vi "Custom VISA Init Selector.vi"(5 "Interface filter (all)":T1={"GPIB"=TRUE, "Serial"=TRUE, "TCP"=TRUE, "USB"=TRUE}, 7 "Initial enumerate? (False)":bool, 8 "error in (no error)":errorcluster, 10 "VISA address (Empty)":refnum<visa-resource-name>, 11 "VISA menu ref":refnum<vi>) -> (0 "error out":errorcluster)   [LabVIEW 2020, in "Get COM Descriptor.lvlib"]
doc: "Call this to initialize custom VISA Ring control at start of panel. It will make initial menu with \"Refresh\" option. If you pass in VISA, it will make default item from the VISA address. Otherwise it will use Ring.Text as default.\nOptionally does initial VISA enumeration to fill in the Ring.\n\nDetails: https://github.com/smaslan/get-com-descriptor"
uses:
  Get COM Descriptor.lvlib
  Custom VISA Filters.ctl
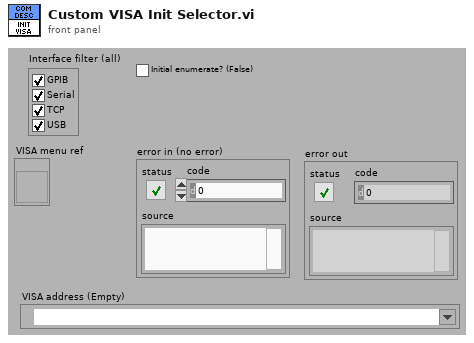
[diagram p1: front panel]
types:
  T1 = typedef "Get COM Descriptor.lvlib/Custom VISA Filters.ctl" = cluster{"GPIB":bool, "Serial":bool, "TCP":bool, "USB":bool}
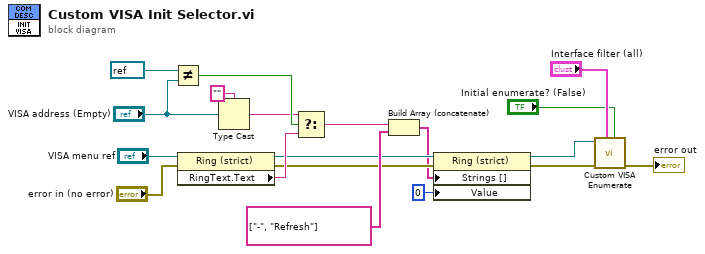
[diagram p0: block diagram]
diagram:
  n1 = Not Equal?(x=refnum<visa-resource-name> refnum ("reference"), y="VISA address (Empty)") -> (x != y?=w13:bool)
  n2 = property class="Ring (strict)"(reference="VISA menu ref", error in="error in (no error)") -> (reference out=w10:refnum<vi>, error out=w9:errorcluster, "RingText.Text"=w11:string)
  n3 = Type Cast(type="", x="VISA address (Empty)") -> (*(type *) &x=w12:string)
  n4 = Select(t=w12, s=w13, f=w11) -> (s? t:f=w7:string)
  n5 = Build Array (concatenate)(w7, string[] ["-", "Refresh"] ("Strings []")) -> (w8:string[])
  n6 = property class="Ring (strict)"(reference=w10, error in=w9, "Strings []"=w8, "Value"=u16 0) -> (reference out=w3:refnum<vi>, error out=w5:errorcluster)
  n7 = call "Custom VISA Enumerate.vi"("Force refresh? (False)"="Initial enumerate? (False)", "Interface filter (all)"="Interface filter (all)", "error in (no error)"=w5, "VISA menu ref"=w3) -> ("error out"=→"error out":errorcluster)  [unwired: 5 in, 2 out]
